vi "GUI_Test_For_Main_Code.vi"() -> ()   [LabVIEW 2018]
uses:
  Type_Def_Current_state_output.ctl
panel:
  out "currentState":T1
  in  "Vent":bool
  in  "SystemCheck":bool
  in  "Shutdown":bool
  in  "ServicePush":bool
  in  "Service":bool
  in  "Ready":bool
  in  "Launch":bool
  in  "IsPowered":bool
  in  "ForceIdle":bool
  in  "Fault":bool
  in  "Stop Button":bool
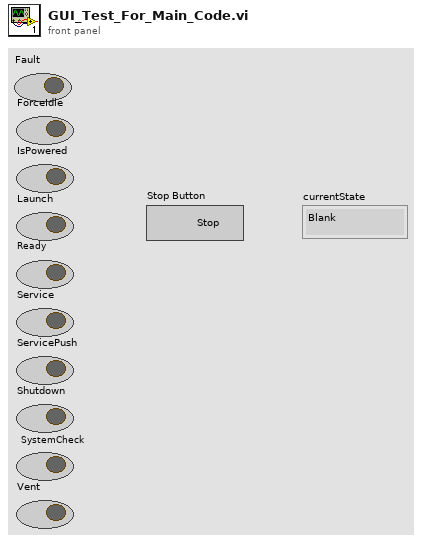
[diagram p1: front panel]
types:
  T1 = typedef "Type_Def_Current_state_output.ctl" = enum16{"Blank", "Systems Check", "Idle", "Ready", "Pushing", "CrawlingPrecharge", "Braking", "Fault", "Boot Up", "Unpowered", "Crawling", "Shutdown", "Service Push", "Service Wait", "Vent", "Precharge", "Cooldown"}
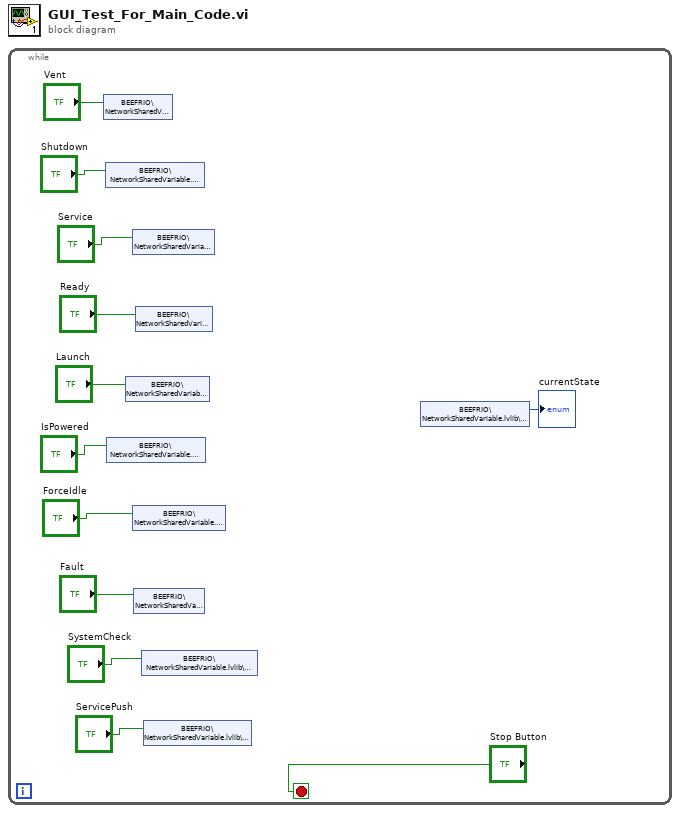
[diagram p0: block diagram]
diagram:
  n1 = while {
    stop <- "Stop Button" stop-if-true
    n2 = shared-variable "BEEFRIO\\NetworkSharedVariable.lvlib\\Vent"("Vent") -> ()  [unwired: 1 in, 1 out]
    n3 = shared-variable "BEEFRIO\\NetworkSharedVariable.lvlib\\Shutdown"("Shutdown") -> ()  [unwired: 1 in, 1 out]
    n4 = shared-variable "BEEFRIO\\NetworkSharedVariable.lvlib\\IsPowered"("IsPowered") -> ()  [unwired: 1 in, 1 out]
    n5 = shared-variable "BEEFRIO\\NetworkSharedVariable.lvlib\\Launch"("Launch") -> ()  [unwired: 1 in, 1 out]
    n6 = shared-variable "BEEFRIO\\NetworkSharedVariable.lvlib\\Service"("Service") -> ()  [unwired: 1 in, 1 out]
    n7 = shared-variable "BEEFRIO\\NetworkSharedVariable.lvlib\\ForceIdle"("ForceIdle") -> ()  [unwired: 1 in, 1 out]
    n8 = shared-variable "BEEFRIO\\NetworkSharedVariable.lvlib\\Fault"("Fault") -> ()  [unwired: 1 in, 1 out]
    n9 = shared-variable "BEEFRIO\\NetworkSharedVariable.lvlib\\Ready"("Ready") -> ()  [unwired: 1 in, 1 out]
    n10 = shared-variable "BEEFRIO\\NetworkSharedVariable.lvlib\\SystemCheck"("SystemCheck") -> ()  [unwired: 1 in, 1 out]
    n11 = shared-variable "BEEFRIO\\NetworkSharedVariable.lvlib\\ServicePush"("ServicePush") -> ()  [unwired: 1 in, 1 out]
    n12 = shared-variable "BEEFRIO\\NetworkSharedVariable.lvlib\\currentState"() -> (→"currentState":T1)  [unwired: 1 in, 1 out]
  }
